vi "Select_a_Channel.vi"(6 "Mode":T1(ring), 7 "Extra channel names":string[](array[string]), 8 "Data Filename":path) -> (0 "Current Values":string[](array[string]), 1 "Channel Values":string[](array[string]), 2 "Selected Channel Names":string[](array[string]), 3 "Data Filename Out":path)   [LabVIEW 2012]
uses:
  ADAM Client/Sub VIs/ADAM Controls/Channel_names.ctl
  ADAM Client/Sub VIs/ADAM Controls/Calib_type_ADAM.ctl
panel:
  in  "Tolerance":dbl=1.0 format="%.4f"
  in  "OK":bool
  in  "Search String":string
  in  "Listbox":i32[](listbox)
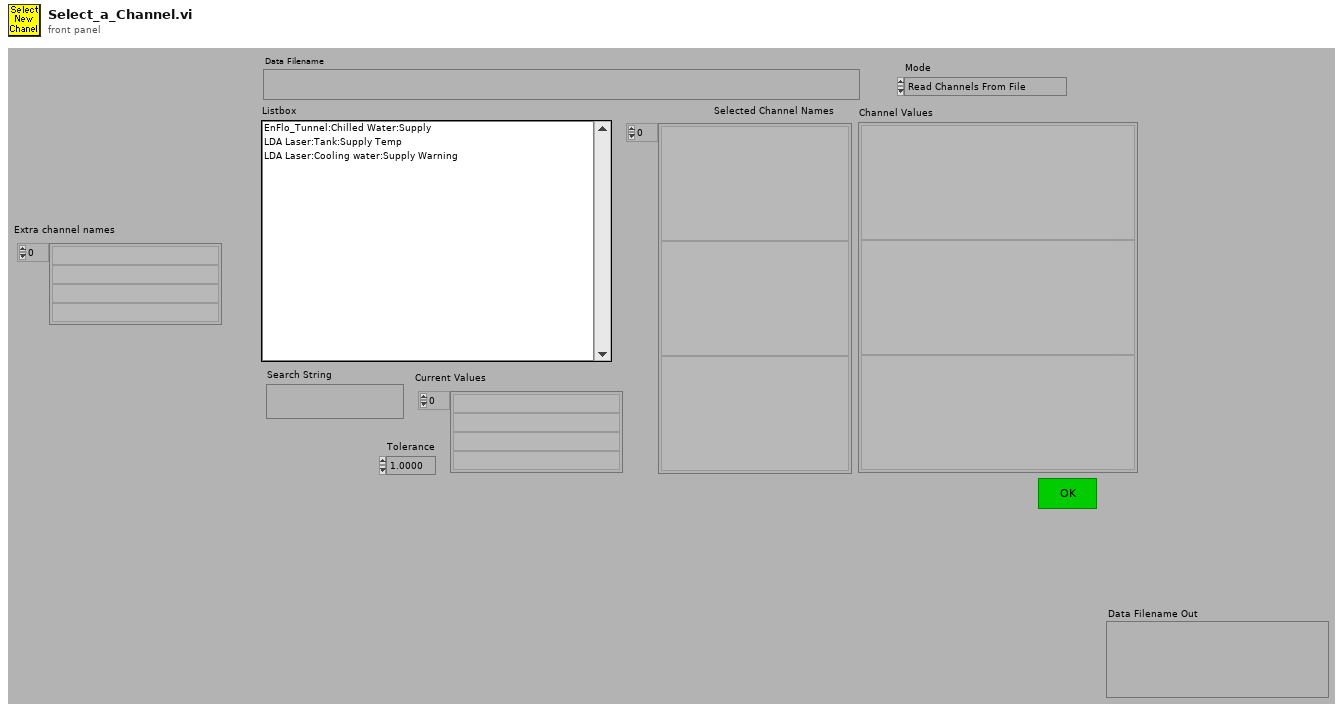
[diagram p1: front panel]
types:
  T1 = enum16{"Read Channels From File", "Read Channels from Server"}
  T2 = typedef "Channel_names.ctl" = enum16{"Active Only", "Active + Off", "All Channels"}
  T3 = typedef "Calib_type_ADAM.ctl" = enum16{"Raw", "Bx + A", "Cx^2 + Bx + A", "Dx^3 + Cx^2 + Bx + A", "In Band", "Hi-Tec Q", "Hi-Tec M_dot", "Text"}
  T4 = enum32{"existing file", "new file", "new or existing file", "existing dir", "new dir", "new or existing dir", "existing file (use LLBs)", "new file (use LLBs)", "new or existing file (use LLBs)", "new or existing file or directory (use LLBs)"}
  T5 = typedef "Ch_description_ADAM.ctl" = cluster{"Ch Name":string, "Type":T6, "Function":T7, "Ch State":T8, "Calibration type":T3, "A":dbl, "B":dbl, "C":dbl, "D":dbl, "Comments":string, "Address":T9, "String":string, "Duty":u16}
  T6 = typedef "Module_type_ADAM.ctl" = string
  T7 = typedef "Function_ADAM.ctl" = enum16{"Analogue Input", "Digital Input", "Event counter", "Event rate", "Analogue Output", "Digital Output", "Relay Output"}
  T8 = typedef "Channel_State.ctl" = enum16{"On", "Off", "Always On", "Always Off"}
  T9 = typedef "Address.ctl" = cluster{"Main":i32, "Ch.":i32, "Sub":i32, "Port Name":string}
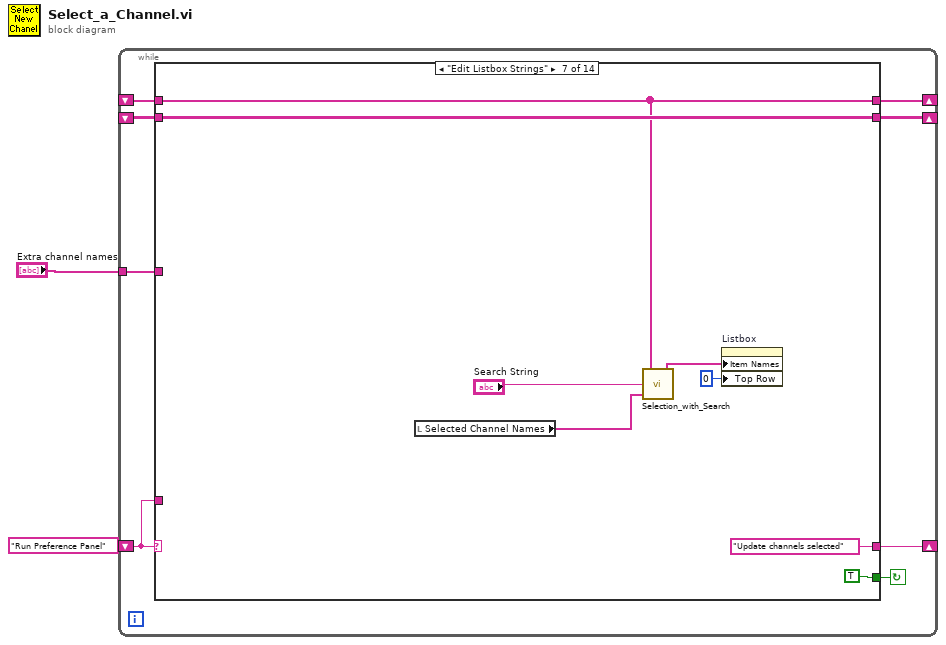
[diagram p0: block diagram]
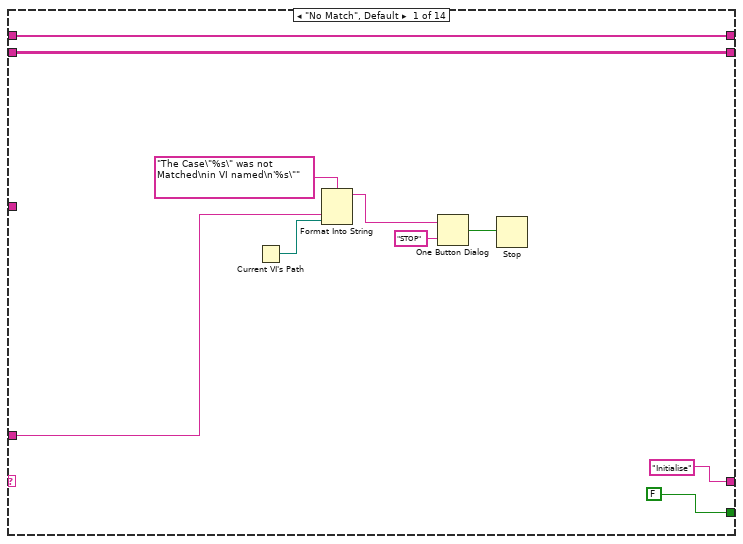
[diagram p2: hidden frame]
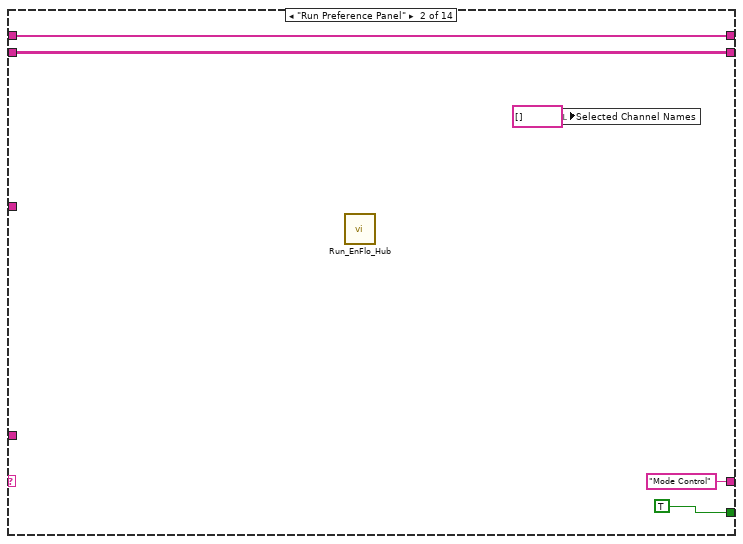
[diagram p3: hidden frame]
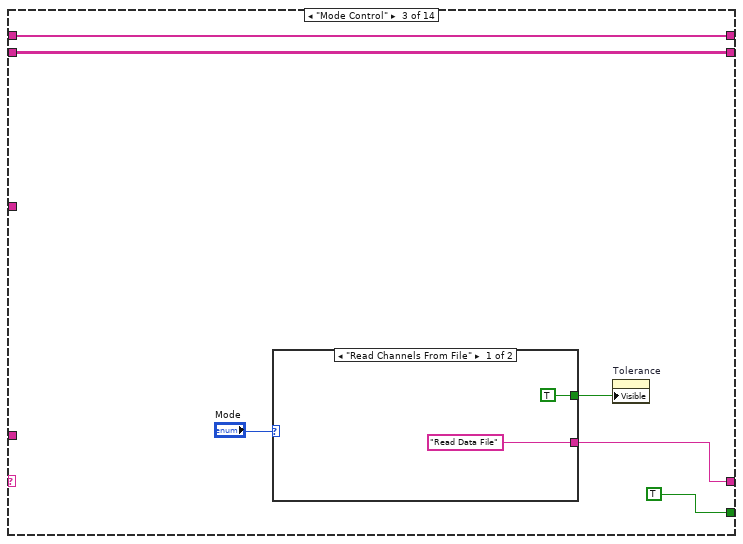
[diagram p4: hidden frame]
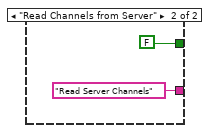
[diagram p5: hidden frame]
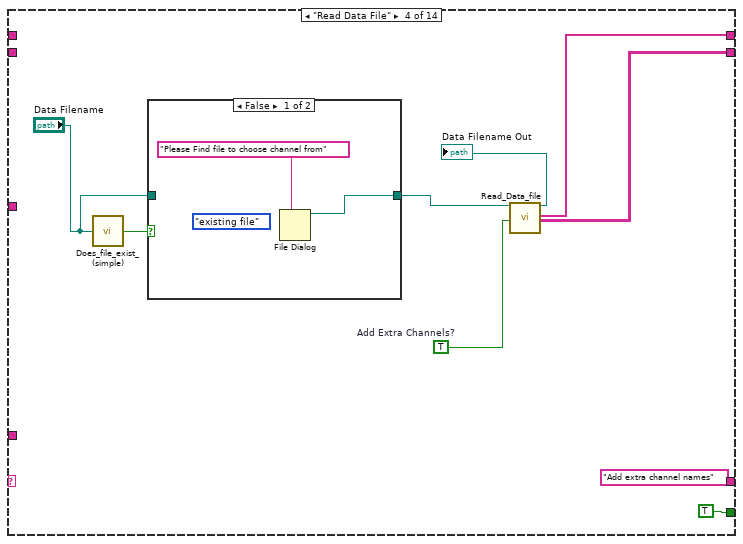
[diagram p6: hidden frame]
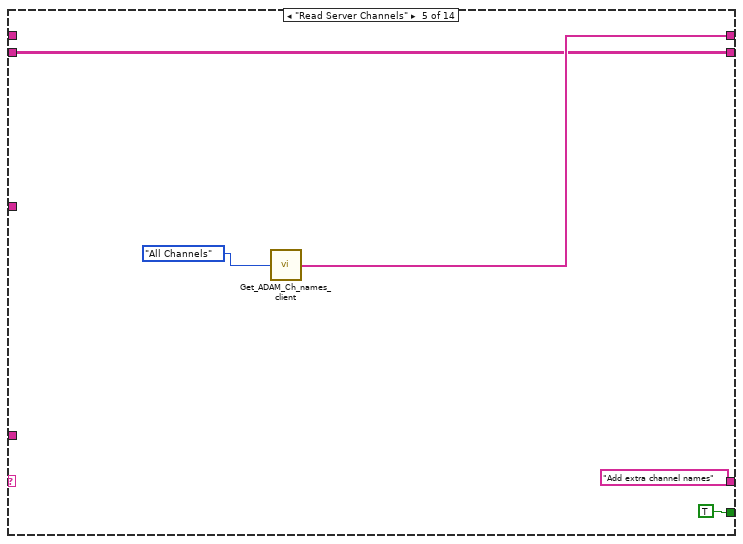
[diagram p8: hidden frame]
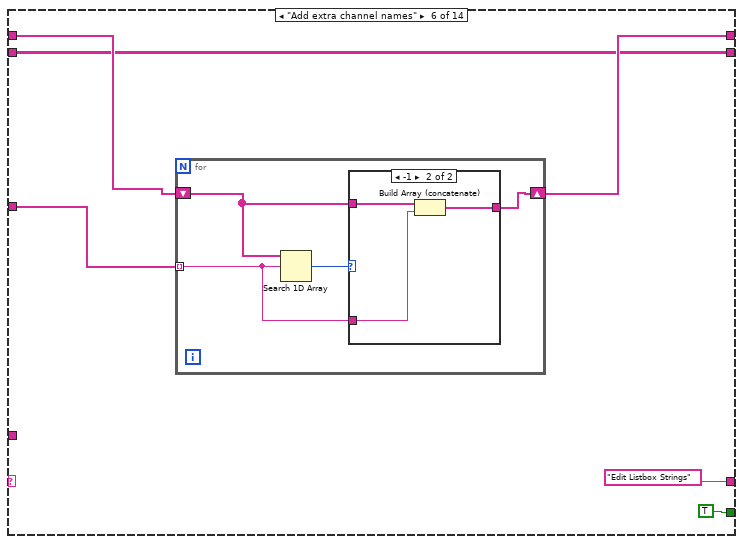
[diagram p9: hidden frame]
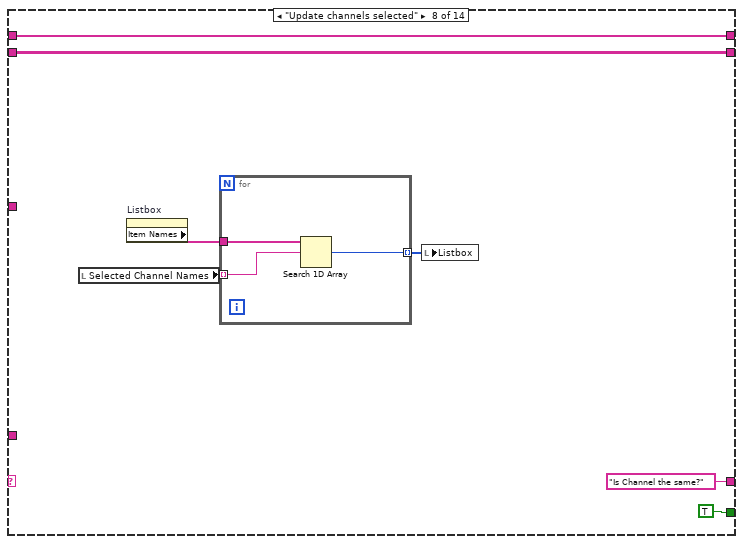
[diagram p11: hidden frame]
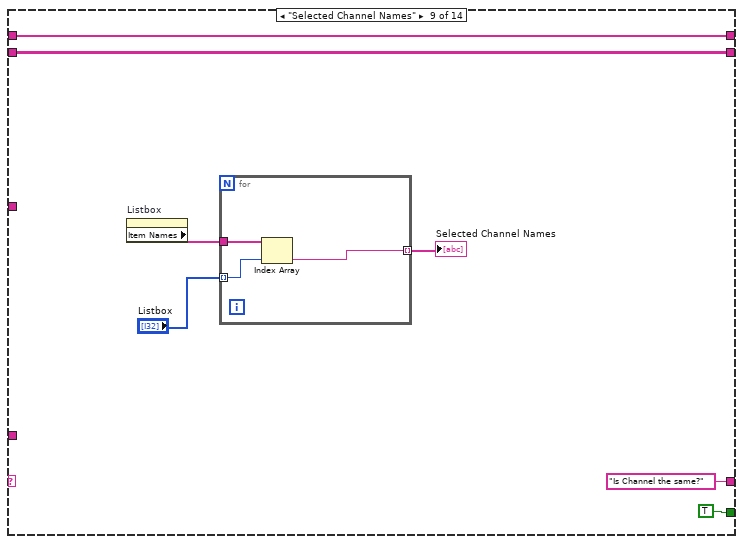
[diagram p12: hidden frame]
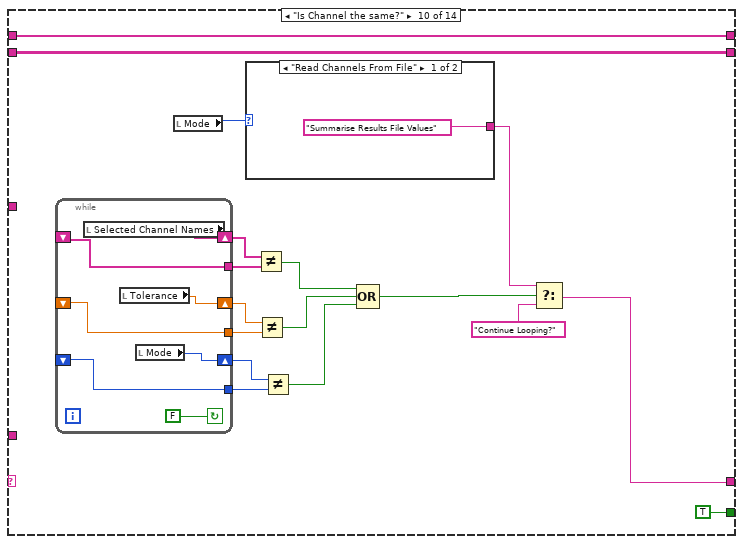
[diagram p13: hidden frame]
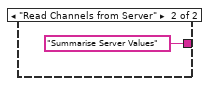
[diagram p14: hidden frame]
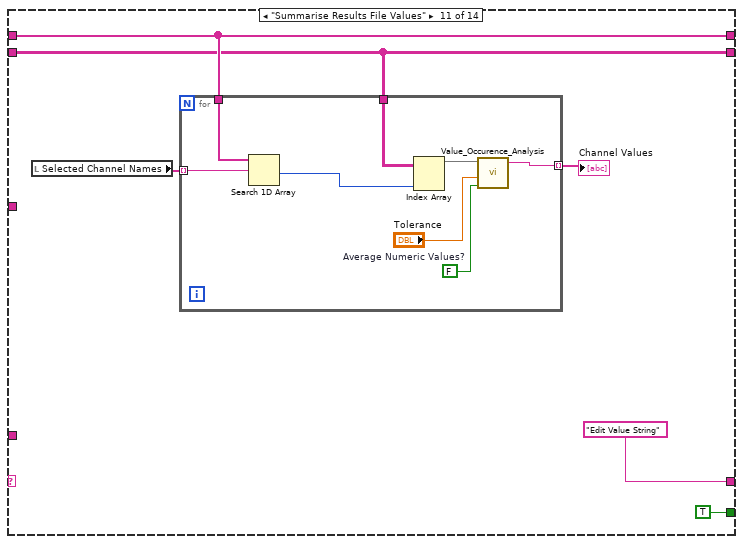
[diagram p15: hidden frame]
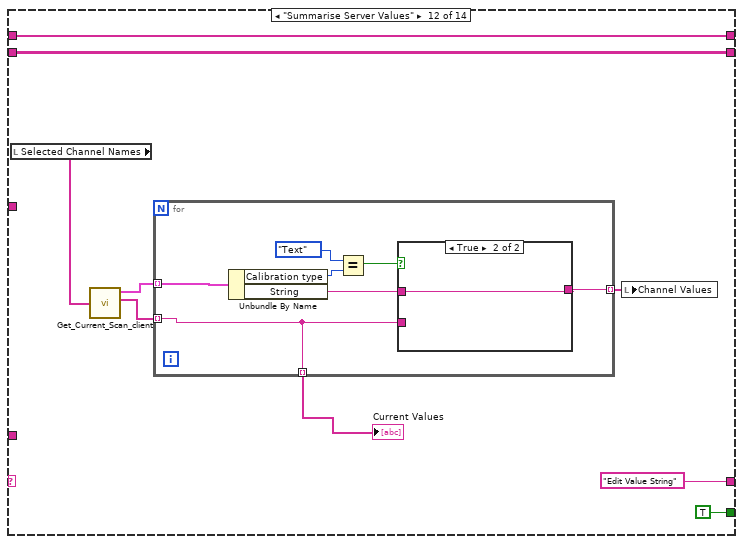
[diagram p16: hidden frame]
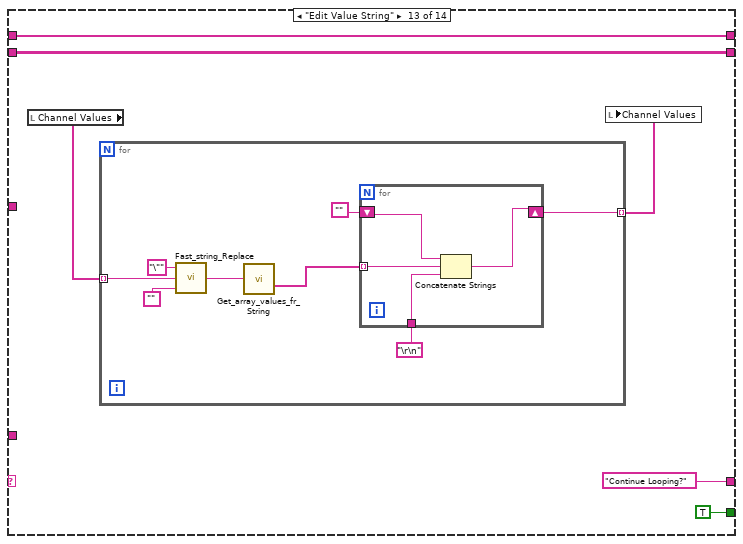
[diagram p18: hidden frame]
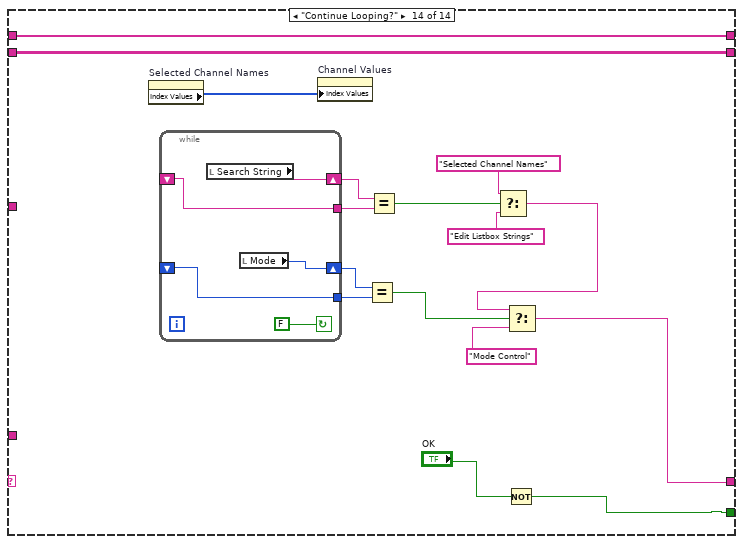
[diagram p19: hidden frame]
diagram:
  n1 = while {
    shift-left: _ -> [w4]
    shift-right: [w6] -> _
    shift-left: _ -> [w5]
    shift-right: [w7] -> _
    shift-left: "Run Preference Panel" -> [w8]
    shift-right: [w9] -> _
    tunnel: "Extra channel names" -> [w3]
    stop <- w10 continue-if-true
    n2 = case shown="\"Edit Listbox Strings\"" w8 {
      tunnel: [FALSE TRUE TRUE TRUE TRUE TRUE TRUE TRUE TRUE TRUE TRUE TRUE TRUE w183] -> w10
      tunnel: ["Initialise" "Mode Control" w28 "Add extra channel names" "Add extra channel names" "Edit Listbox Strings" "Update channels selected" "Is Channel the same?" "Is Channel the same?" w106 "Edit Value String" "Edit Value String" "Continue Looping?" w178] -> w9
      tunnel: w8 -> [w15 _ _ _ _ _ _ _ _ _ _ _ _ _]
      tunnel: [w12 w24 w30 w42 w50 w54 w72 w79 w89 w109 w125 w140 w155 w186] -> w7
      tunnel: [w11 w23 w29 w41 w49 w53 w73 w80 w90 w110 w123 w141 w156 w185] -> w6
      tunnel: w5 -> [w12 w24 w30 _ _ w56 w72 w79 w89 w109 w125 w140 w155 w186]
      tunnel: w4 -> [w11 w23 w29 _ w49 w53 w73 w80 w90 w110 w123 w141 w156 w185]
      tunnel: w3 -> [_ _ _ _ _ w55 _ _ _ _ _ _ _ _]
      frame "No Match", Default {
        n3 = Current VI's Path() -> (path=w14:path)
        n4 = Format Into String(format string="The Case\"%s\" was not Matched\nin VI named\n'%s\"" ("Format String"), w15, w14) -> (resulting string=w18:string)  [unwired: 2 in, 1 out]
        n5 = One Button Dialog(message=w18, button name ("OK")="STOP") -> (true=w16:bool)
        n6 = Stop(stop? (T)=w16) -> ()
      }
      frame "Run Preference Panel" {
        n7 = call "Run_EnFlo_Hub.vi"() -> ()  [unwired: 8 out]
        n8 = local write "Selected Channel Names"(string[] [] ("Selected Channel Names")) -> ()
      }
      frame "Mode Control" {
        n9 = case shown="\"Read Channels From File\"" "Mode" {
          tunnel: ["Read Data File" "Read Server Channels"] -> w28
          tunnel: [TRUE FALSE] -> w27
          frame "Read Channels From File" {
          }
          frame "Read Channels from Server" {
          }
        }
        n10 = property on="Tolerance" class="DigNum (strict)"("Visible"=w27) -> ()  [unwired: 2 in, 2 out]
      }
      frame "Read Data File" {
        w40 = TRUE  # Add Extra Channels?
        n11 = call "Does_file_exist_(simple).vi"("Pathname"="Data Filename") -> ("exists?"=w39:bool)
        n12 = case shown="False" w39 {
          tunnel: [w46 w47] -> w37
          tunnel: "Data Filename" -> [_ w47]
          frame False {
            (unwired) T4."existing file" ("select mode (2)")
            n13 = File Dialog(7:"Please Find file to choose channel from" ("prompt")) -> (3:w46:path)  [unwired: 1 in, 8 out]
          }
          frame True {
          }
        }
        n14 = call "Read_Data_file.vi"("Results file"=w37, "Add Extra Channels?"=w40) -> ("Results file Out"=→"Data Filename Out":path, "Ch names Out"=w42:string[], "Channel Values Out"=w41:string[][])  [unwired: 3 in, 12 out]
      }
      frame "Read Server Channels" {
        n15 = call "Get_ADAM_Ch_names_client.vi"("Channel names set"=Channel_names."All Channels") -> ("Ch names"=w50:string[])
      }
      frame "Add extra channel names" {
        n16 = for {
          shift-right: [w60] -> w54
          shift-left: w56 -> [w61]
          tunnel: w55 -> [w59] mode=indexing
          n17 = Search 1D Array(1D array=w61, element=w59) -> (index of element=w62:i32)  [unwired: 1 out]
          n18 = case shown="-1" w62 {
            tunnel: w61 -> [w63 w66]
            tunnel: [w63 w65] -> w60
            tunnel: w59 -> [_ w64]
            frame 0, Default {
            }
            frame -1 {
              n19 = Build Array (concatenate)(w66, w64) -> (w65:string[])
            }
          }
        }
      }
      frame "Edit Listbox Strings" {
        n20 = local read "Selected Channel Names"() -> (w68:string[])
        n21 = call "Selection_with_Search.vi"("Selected Channel Names"=w68, "Search String"="Search String", "All Channel Names"=w72) -> ("Item Names"=w69:string[])
        n22 = property on="Listbox" class="LstBox (strict)"("Item Names"=w69, "Top Row"=0) -> ()  [unwired: 2 in, 2 out]
      }
      frame "Update channels selected" {
        n23 = local read "Selected Channel Names"() -> (w76:string[])
        n24 = property on="Listbox" class="LstBox (strict)"() -> ("Item Names"=w77:string[])  [unwired: 2 in, 2 out]
        n25 = for {
          tunnel: w77 -> [w84]
          tunnel: w76 -> [w83] mode=indexing
          tunnel: [w82] -> w75 mode=indexing
          n26 = Search 1D Array(1D array=w84, element=w83) -> (index of element=w82:i32)  [unwired: 1 out]
        }
        n27 = local write "Listbox"(w75) -> ()
      }
      frame "Selected Channel Names" {
        n28 = property on="Listbox" class="LstBox (strict)"() -> ("Item Names"=w87:string[])  [unwired: 2 in, 2 out]
        n29 = for {
          tunnel: w87 -> [w94]
          tunnel: "Listbox" -> [w93] mode=indexing
          tunnel: [w92] -> w85 mode=indexing
          n30 = Index Array(array=w94, index=w93) -> (element=w92:string)
        }
        "Selected Channel Names" <- w85
      }
      frame "Is Channel the same?" {
        n31 = while {
          tunnel: [w114] -> w98
          shift-left: _ -> [w114]
          shift-right: [w113] -> w99
          tunnel: [w115] -> w105
          shift-left: _ -> [w115]
          shift-right: [w116] -> w104
          tunnel: [w117] -> w107
          shift-left: _ -> [w117]
          shift-right: [w118] -> w108
          stop <- FALSE continue-if-true
          n32 = local read "Selected Channel Names"() -> (w118:string[])
          n33 = local read "Tolerance"() -> (w116:dbl)
          n34 = local read "Mode"() -> (w113:T1)
        }
        n35 = local read "Mode"() -> (w100:T1)
        n36 = case shown="\"Read Channels From File\"" w100 {
          tunnel: ["Summarise Results File Values" "Summarise Server Values"] -> w96
          frame "Read Channels From File" {
          }
          frame "Read Channels from Server" {
          }
        }
        n37 = Not Equal?(x=w108, y=w107) -> (x != y?=w103:bool)
        n38 = Not Equal?(x=w104, y=w105) -> (x != y?=w102:bool)
        n39 = Not Equal?(x=w99, y=w98) -> (x != y?=w97:bool)
        n40 = Compound Arithmetic op=OR(w103, w102, w97) -> (w101:bool)
        n41 = Select(t=w96, s=w101, f="Continue Looping?") -> (s? t:f=w106:string)
      }
      frame "Summarise Results File Values" {
        n42 = local read "Selected Channel Names"() -> (w124:string[])
        n43 = for {
          tunnel: w125 -> [w134]
          tunnel: w124 -> [w133] mode=indexing
          tunnel: w123 -> [w131]
          tunnel: [w128] -> w121 mode=indexing
          w127 = FALSE  # Average Numeric Values?
          n44 = Search 1D Array(1D array=w134, element=w133) -> (index of element=w132:i32)  [unwired: 1 out]
          n45 = Index Array(array=w131, index (col)=w132) -> (element=w130:string[])  [unwired: 1 in]
          n46 = call "Value_Occurence_Analysis.vi"("Average Numeric Values?"=w127, "Tolerance"="Tolerance", "String Array"=w130) -> ("Output String"=w128:string)  [unwired: 1 in, 2 out]
        }
        "Channel Values" <- w121
      }
      frame "Summarise Server Values" {
        n47 = local read "Selected Channel Names"() -> (w139:string[])
        n48 = call "Get_Current_Scan_client.vi"("ADAM Ch Names"=w139) -> ("Ch Description Array"=w138:T5[], "String values"=w137:string[])  [unwired: 2 out]
        n49 = for {
          tunnel: w138 -> [w145] mode=indexing
          tunnel: w137 -> [w144] mode=indexing
          tunnel: [w146] -> w135 mode=indexing
          tunnel: [w144] -> w136 mode=indexing
          n50 = Unbundle By Name(w145) -> ("Calibration type"=w150:T3, "String"=w147:string)
          n51 = Equal?(x=Calib_type_ADAM."Text" ("Calibration Type"), y=w150) -> (x = y?=w148:bool)
          n52 = case shown="True" w148 {
            tunnel: [w151 w152] -> w146
            tunnel: w147 -> [_ w152]
            tunnel: w144 -> [w151 _]
            frame False {
            }
            frame True {
            }
          }
        }
        "Current Values" <- w136
        n53 = local write "Channel Values"(w135) -> ()
      }
      frame "Edit Value String" {
        n54 = local read "Channel Values"() -> (w154:string[])
        n55 = for {
          tunnel: w154 -> [w160] mode=indexing
          tunnel: [w159] -> w153 mode=indexing
          n56 = call "Fast_string_Replace.vi"("Replace match with:"="", "Input String"=w160, "regular expression"="\"") -> ("Output String"=w161:string)  [unwired: 2 out]
          n57 = call "Get_array_values_fr_String.vi"("String Value"=w161) -> ("String array"=w166:string[])  [unwired: 1 out]
          n58 = for {
            shift-right: [w167] -> w159
            shift-left: "" -> [w170]
            tunnel: w166 -> [w169] mode=indexing
            tunnel: "\r\n" -> [w168]
            n59 = Concatenate Strings(w170, w169, w168) -> (w167:string)
          }
        }
        n60 = local write "Channel Values"(w153) -> ()
      }
      frame "Continue Looping?" {
        n61 = property on="Selected Channel Names" class="Arr (strict)"() -> ("Index Values"=w171:u32[])  [unwired: 2 in, 2 out]
        n62 = while {
          tunnel: [w188] -> w177
          shift-left: _ -> [w188]
          shift-right: [w189] -> w176
          tunnel: [w191] -> w181
          shift-left: _ -> [w191]
          shift-right: [w190] -> w182
          stop <- FALSE continue-if-true
          n63 = local read "Search String"() -> (w189:string)
          n64 = local read "Mode"() -> (w190:T1)
        }
        n65 = property on="Channel Values" class="Arr (strict)"("Index Values"=w171) -> ()  [unwired: 2 in, 2 out]
        n66 = Equal?(x=w182, y=w181) -> (x = y?=w180:bool)
        n67 = Equal?(x=w176, y=w177) -> (x = y?=w175:bool)
        n68 = Select(t="Selected Channel Names", s=w175, f="Edit Listbox Strings") -> (s? t:f=w172:string)
        n69 = Not(x="OK") -> (.not. x?=w183:bool)
        n70 = Select(t=w172, s=w180, f="Mode Control") -> (s? t:f=w178:string)
      }
    }
  }
